vi "SpeedTest.vi"() -> ()   [LabVIEW 2009]
panel:
  out "x-y":dbl
  out "x/y":dbl
  out "Waveform Graph":dbl[](graph)
  in  "A/D Channel":dbl
  # "This LabVIEW item is deprecated.\n\nIt is believed to be unused and will be removed in a future version of SRV."
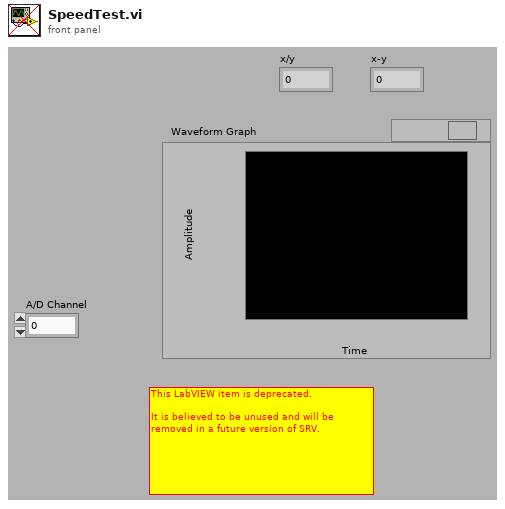
[diagram p1: front panel]
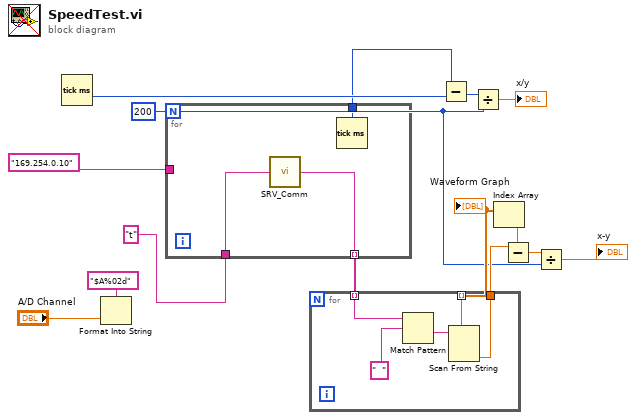
[diagram p0: block diagram]
diagram:
  w3 = 200
  n1 = Tick Count (ms)() -> (millisecond timer value=w13:u32)
  n2 = Format Into String(format string="$A%02d" ("Command Sent"), "A/D Channel") -> ()  [unwired: 2 in, 2 out]
  n3 = for {
    N: w3 -> [_]
    tunnel: "t" ("Command Sent") -> [w17]
    tunnel: [w16] -> w9 mode=indexing
    tunnel: [w18] -> w8
    tunnel: "169.254.0.10" ("IP address") -> [_]
    n4 = call "SRV_Comm.vi"("Command Sent"=w17) -> ("Reply"=w16:string)  [unwired: 2 in, 2 out]
    n5 = Tick Count (ms)() -> (millisecond timer value=w18:u32)
  }
  n6 = for {
    tunnel: w9 -> [w20] mode=indexing
    tunnel: [w19] -> w6 mode=indexing
    tunnel: [w19] -> w7
    n7 = Match Pattern(string=w20, regular expression="  " ("Command Sent")) -> (after substring=w21:string)  [unwired: 1 in, 3 out]
    n8 = Scan From String(input string=w21) -> (output 1=w19:dbl)  [unwired: 4 in, 3 out]
  }
  "Waveform Graph" <- w6
  n9 = Subtract(x=w8, y=w13) -> (x-y=w12:u32)
  n10 = Divide(x=w12, y=w3) -> (x/y=→"x/y":dbl)
  n11 = Index Array(array=w6) -> (element=w5:dbl)  [unwired: 1 in]
  n12 = Subtract(x=w7, y=w5) -> (x-y=w4:dbl)
  n13 = Divide(x=w4, y=w3) -> (x/y=→"x-y":dbl)
